vi "Get VI Info.vi"(6 "Error In":errorcluster, 8 "VI Path":path, 9 "App Ref":refnum<vi>) -> (0 "Error Out":errorcluster, 3 "VI Info":T1 {"TimeStamp" format="%<%x %.3X>T"})   [LabVIEW 2018]
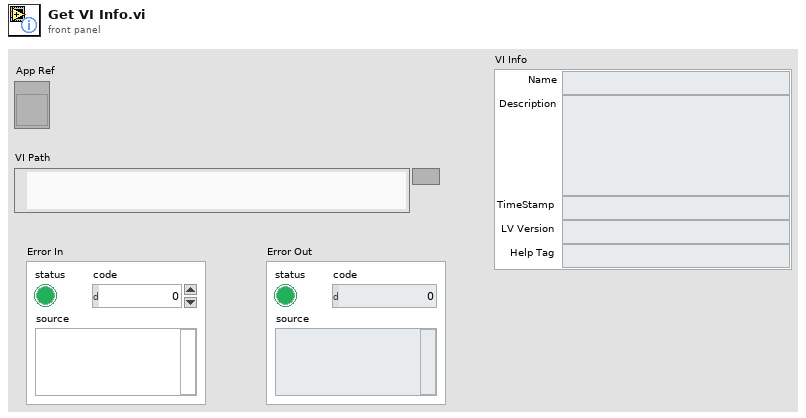
[diagram p1: front panel]
types:
  T1 = cluster{"Name":string, "Description":string, "TimeStamp":timestamp, "LV Version":string, "Help Tag":string}
  T2 = typedef "Librarian File Info Out.ctl" = cluster{"creation date":u32, "last mod date":u32, "type":string, "creator":string, "LV version":i32, "size":i32, "top level":bool}
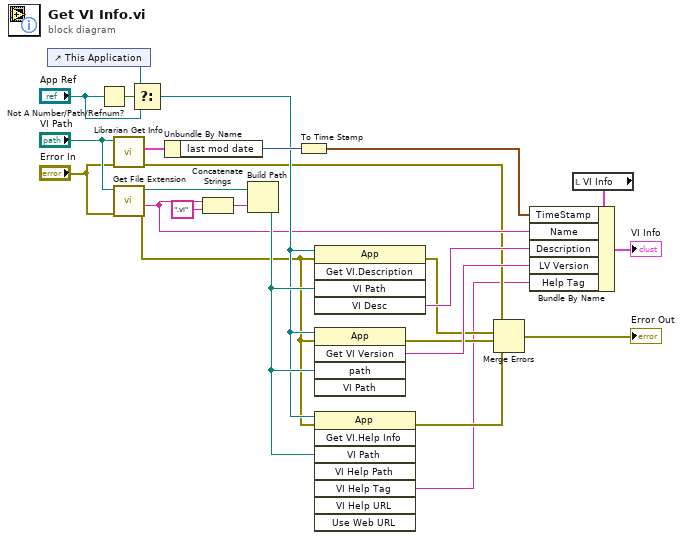
[diagram p0: block diagram]
diagram:
  n1 = control-ref of="This Application"() -> (w13:refnum<vi>)
  n2 = Not A Number/Path/Refnum?(number/path/refnum="App Ref") -> (NaN/Path/Refnum?=w14:bool)
  n3 = call <vilib>:"Librarian Get Info.vi"("error in (no error)"="Error In", "path"="VI Path") -> ("error out"=w8:errorcluster, "file information"=w17:T2)  [unwired: 7 in, 1 out]
  n4 = call <vilib>:"Get File Extension.vi"("error in (no error)"="Error In", "file"="VI Path") -> ("error out"=w10:errorcluster, "filename without extension"=w9:string, "dup file"=w25:path)  [unwired: 5 in, 2 out]
  n5 = Select(t=w13, s=w14, f="App Ref") -> (s? t:f=w11:refnum<vi>)
  n6 = Unbundle By Name(w17) -> ("last mod date"=w16:u32)
  n7 = Concatenate Strings(w9, ".vi" ("string")) -> (w24:string)
  n8 = Build Path(base path=w25, name or relative path=w24) -> (appended path=w18:path)
  n9 = To Time Stamp(1:w16) -> (0:w3:timestamp)
  n10 = invoke on="Invoke Node" class="App" method="Get VI.Description"(reference=w11, error in=w10, "VI Path"=w18) -> (error out=w7:errorcluster, "VI Desc"=w20:string)  [unwired: 2 in, 3 out]
  n11 = invoke on="Invoke Node" class="App" method="Get VI Version"(reference=w11, error in=w10, "path"=w18) -> (error out=w6:errorcluster, "GetVIVers"=w19:string)  [unwired: 2 in, 3 out]
  n12 = invoke on="Invoke Node" class="App" method="Get VI.Help Info"(reference=w11, error in=w10, "VI Path"=w18) -> (error out=w2:errorcluster, "VI Help Tag"=w1:string)  [unwired: 5 in, 6 out]
  n13 = Merge Errors(w8, w7, w6, w2) -> (→"Error Out":errorcluster)
  n14 = local read "VI Info"() -> (w22:T1)
  n15 = Bundle By Name(cluster=w22, "TimeStamp"=w3, "Name"=w9, "Description"=w20, "LV Version"=w19, "Help Tag"=w1) -> (→"VI Info":T1)
